vi "Get Axial Value.vi"(8 "error in (no error)":errorcluster, 10 "Actuate Settings":T1 {"FC2 Measured Value" format="%.3f"; "Lateral Demand" format="%.3f"; "FC1 Measured Value" format="%.3f"; "Axial Demand" format="%.3f"}, 11 "Dual Cylinder Outer Loop Actuator in":refnum<class "Dual Cylinder Outer Loop Actuator.lvclass">) -> (0 "error out":errorcluster, 2 "Axial Control":dbl[unit] format="%.2f", 3 "Dual Cylinder Outer Loop Actuator out":refnum<class "Dual Cylinder Outer Loop Actuator.lvclass">)   [LabVIEW 2015, in "Dual Cylinder Outer Loop Actuator.lvclass"]
uses:
  Dual Cylinder Outer Loop Actuator.lvclass
  Typedefs/Actuate Arguments.ctl
  Dual Cylinder Outer Loop Actuator.lvclass/Dual Cylinder Outer Loop Actuator.ctl
  <vilib>/addons/control/pid/pid.llb/PID (DBL).vi
  <vilib>/addons/control/pid/NI_PID_pid.lvlib
  Calculators/Cylinder To Actuator Forces/Cylinder To Actuator Forces.lvclass
  Typedefs/FAMT Typedefs.lvlib
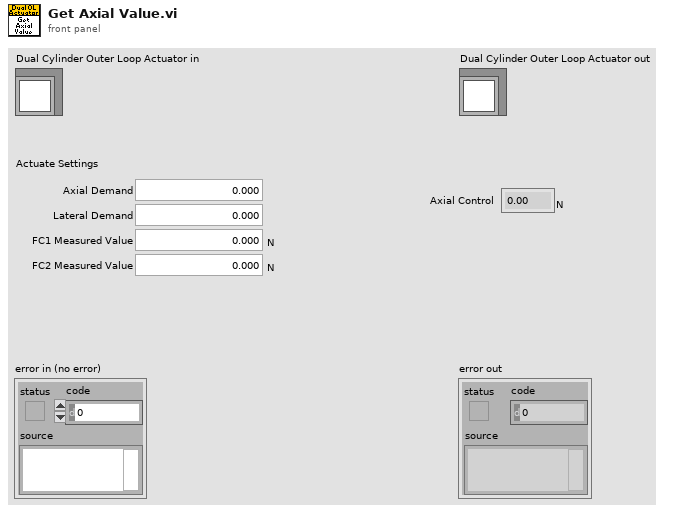
[diagram p1: front panel]
types:
  T1 = typedef "FAMT Typedefs.lvlib/Actuate Arguments.ctl" = cluster{"Axial Demand":dbl, "Lateral Demand":dbl, "FC1 Measured Value":dbl[unit], "FC2 Measured Value":dbl[unit]}
  T2 = cluster{"proportional gain (Kc)":dbl, "integral time (Ti, min)":dbl, "derivative time (Td, min)":dbl}
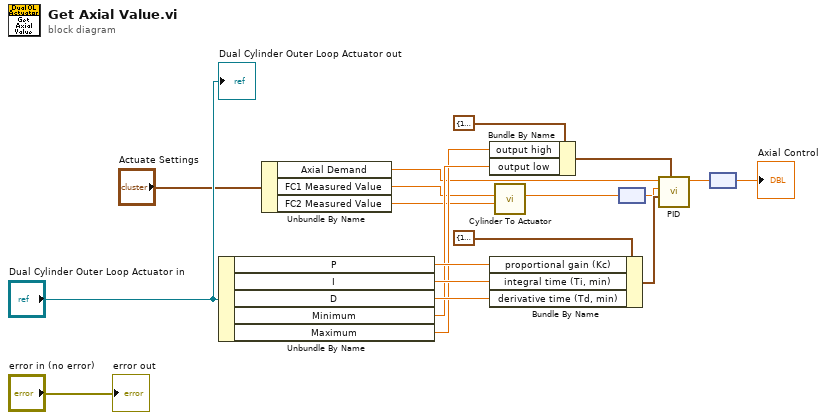
[diagram p0: block diagram]
diagram:
  n1 = Unbundle By Name("Dual Cylinder Outer Loop Actuator in") -> ("P"=w13:dbl, "I"=w12:dbl, "D"=w11:dbl, "Minimum"=w10:dbl, "Maximum"=w9:dbl)
  n2 = Unbundle By Name("Actuate Settings") -> ("Axial Demand"=w4:dbl, "FC1 Measured Value"=w7:dbl[unit], "FC2 Measured Value"=w6:dbl[unit])
  n3 = Bundle By Name(cluster=cluster{"output high":dbl, "output low":dbl} {"output high"=100.0, "output low"=-100.0} ("output range"), "output high"=w9, "output low"=w10) -> (w16:cluster{"output high":dbl, "output low":dbl})
  n4 = Bundle By Name(cluster=T2 {"proportional gain (Kc)"=1.0, "integral time (Ti, min)"=0.01, "derivative time (Td, min)"=0.0} ("PID gains"), "proportional gain (Kc)"=w13, "integral time (Ti, min)"=w12, "derivative time (Td, min)"=w11) -> (w14:T2)
  n5 = call "Cylinder To Actuator.vi"("FC2 Measured Value"=w6, "FC1 Measured Value"=w7) -> ("Axial Force"=w1:dbl[unit])  [unwired: 6 in, 3 out]
  n6 = node(w1) -> (w5:dbl)
  n7 = call-poly <vilib>:"PID.vi"("output range"=w16, "PID gains"=w14, "process variable"=w5, "setpoint"=w4) -> ("output"=w3:dbl)  [unwired: 6 in, 1 out]
  n8 = node(w3) -> (→"Axial Control":dbl[unit])
  "error out" <- "error in (no error)"
  "Dual Cylinder Outer Loop Actuator out" <- "Dual Cylinder Outer Loop Actuator in"
